vi "Prepare Two Step Build.vi"(8 "error in (no error)":errorcluster, 11 "NI_AB_API_DPPL in":refnum<class "NI_AB_API_DPPL.lvclass">) -> (0 "error out":errorcluster, 2 "Build Context":refnum<vi>, 3 "NI_AB_API_DPPL out":refnum<class "NI_AB_API_DPPL.lvclass">)   [LabVIEW 2020, in "NI_AB_API_DPPL.lvclass"]
uses:
  <vilib>/AppBuilder/AB_API/DPPL/NI_AB_API_DPPL.lvclass
  <vilib>/AppBuilder/AB_API/DPPL/NI_AB_API_DPPL.lvclass/NI_AB_API_DPPL.ctl
  <vilib>/AppBuilder/AB_API/PPL/NI_AB_API_PPL.lvclass
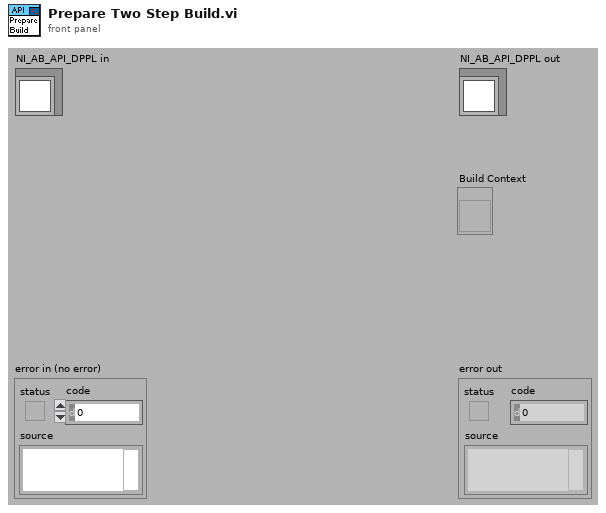
[diagram p1: front panel]
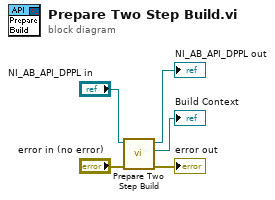
[diagram p0: block diagram]
diagram:
  n1 = call-parent "Prepare Two Step Build.vi"("error in (no error)"="error in (no error)", "NI_AB_API_PPL in"="NI_AB_API_DPPL in") -> ("error out"=→"error out":errorcluster, "Build Context"=→"Build Context":refnum<vi>, "NI_AB_API_PPL out"=→"NI_AB_API_DPPL out":refnum<class "NI_AB_API_DPPL.lvclass">)  [unwired: 7 in]
